vi "BJT_CE_Characterization.vi"() -> ()   [LabVIEW 2020]
panel:
  in  "Tab Control":enum32{"Plot", "Readings", "Information"}(tab)
  out "Temperature / Deg C °":dbl(slide) scale=0.0..100.0
  out "IV Characteristics":cluster{dbl[], dbl[]}[](graph)
  in  "?":bool
  in  "UB":dbl[](array[numeric])=[0.9, 1.0, 1.1, 1.2, 1.3]
  out "UCE":dbl format="%#_3f"
  out "IC":dbl
  out "URC":dbl format="%#_3f"
  out "Numeric":i32
  out "UB/V":dbl
  out "URB/V":dbl format="%#_2f"
  out "UBE/V":dbl format="%#_2f"
  out "UC / V":dbl format="%#_3f"
  out "IB / mA":dbl format="%#_2f"
  # "BJT Values"
  # "IC max = 100 mA"
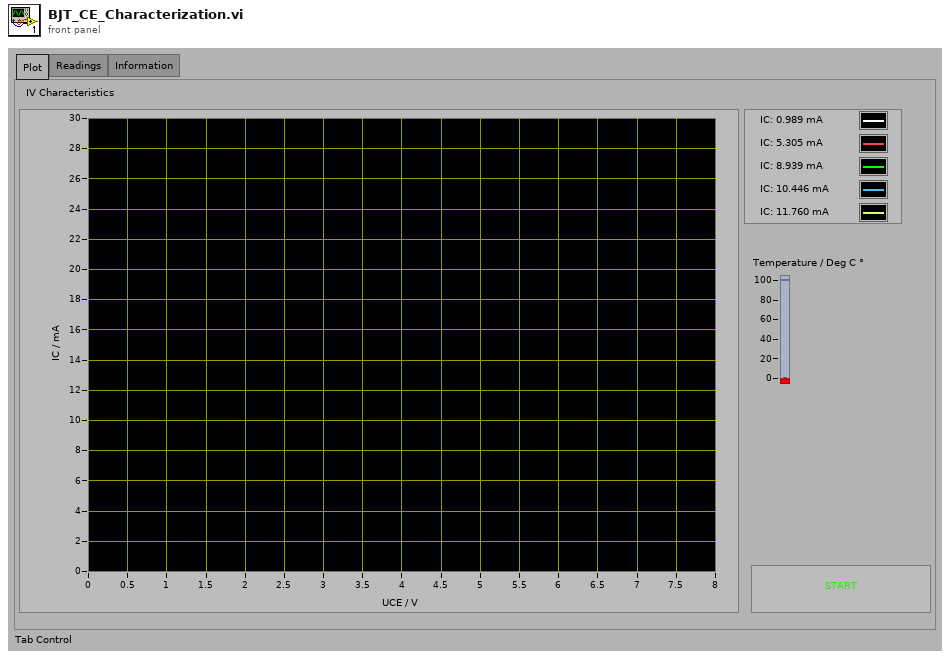
[diagram p1: front panel]
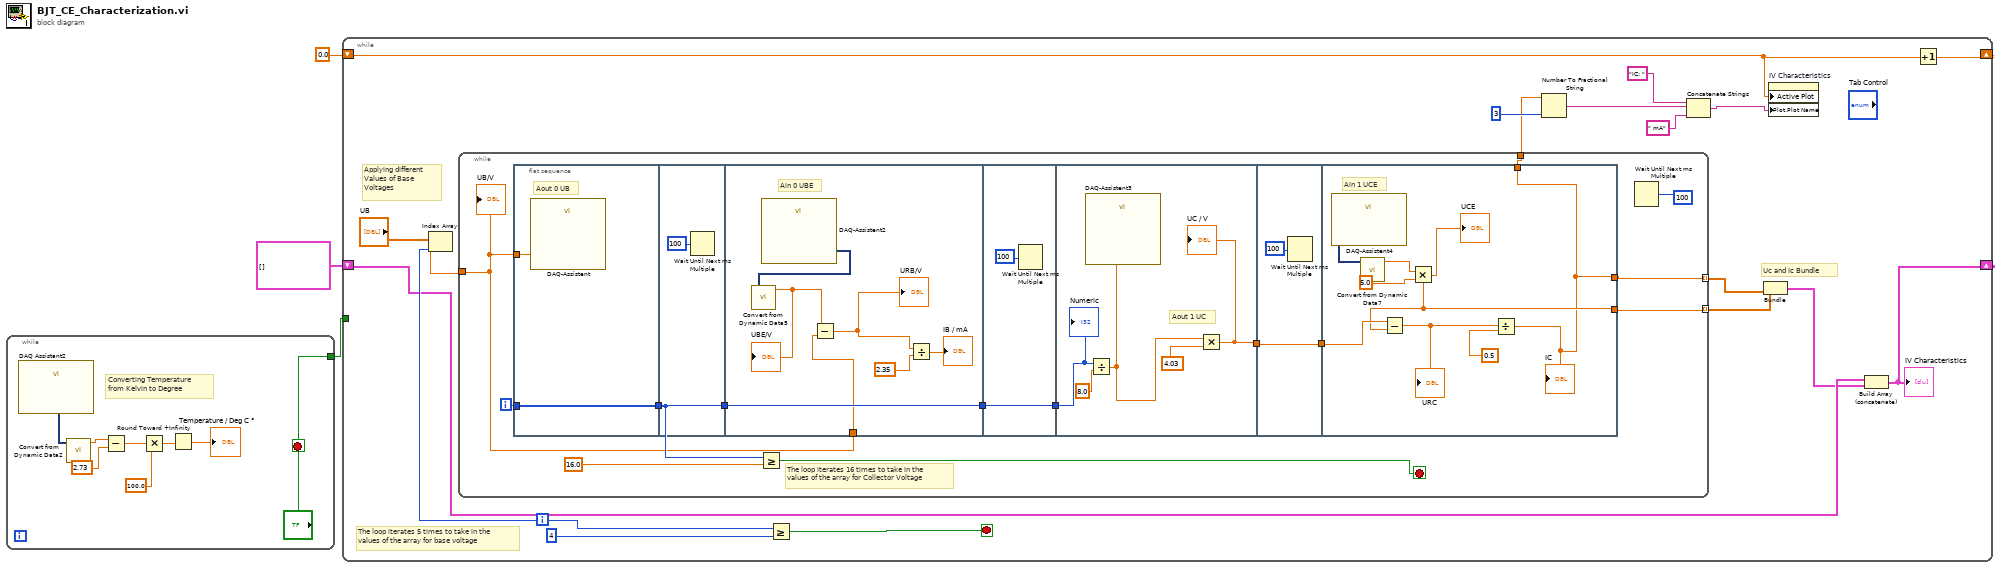
[diagram p0: block diagram]
diagram:
  n1 = while {
    tunnel: ["?"] -> w3
    stop <- "?" stop-if-true
    # "Converting Temperature \nfrom Kelvin to Degree"
    n2 = call "DAQ Assistant2"() -> ("data"=w6:dynamicdata)  [unwired: 17 in, 2 out]
    n3 = call "Convert from Dynamic Data2"("Dynamic Data Type"=w6) -> ("Scalar"=w11:dbl)  [unwired: 3 in]
    n4 = Subtract(x=w11, y=2.73) -> (x-y=w10:dbl)
    n5 = Multiply(x=w10, y=100.0) -> (x*y=w7:dbl)
    n6 = Round Toward +Infinity(x=w7) -> (ceil(x): smallest int >= x=→"Temperature / Deg C °":dbl)
  }
  n7 = while {
    tunnel: w3 -> [_]
    shift-right: [w24] -> _
    shift-left: 0.0 -> [w18]
    shift-right: [w17] -> _
    shift-left: cluster{dbl[], dbl[]}[] [] -> [w16]
    i -> [w27]
    stop <- w28 stop-if-true
    # "Applying different\nValues of Base \nVoltages"
    # "The loop iterates 5 times to take in the \nvalues of the array for base voltage"
    # "Uc and Ic Bundle"
    n8 = Index Array(array="UB", index=w27) -> (element=w29:dbl)
    n9 = while {
      tunnel: w29 -> [w38]
      tunnel: [w36] -> w20
      tunnel: [w35] -> w12 mode=indexing
      tunnel: [w33] -> w13 mode=indexing
      i -> [w41]
      stop <- w43 stop-if-true
      # "The loop iterates 16 times to take in the \nvalues of the array for Collector Voltage"
      n10 = flat-sequence {
        tunnel: w38 -> [w45]
        tunnel: [w44] -> w40
        tunnel: w41 -> [w44]
        tunnel: w40 -> [w47]
        tunnel: [w47] -> w39
        tunnel: w39 -> [w54]
        tunnel: [w54] -> w32
        tunnel: w38 -> [w50]
        tunnel: w32 -> [w56]
        tunnel: [w56] -> w31
        tunnel: w31 -> [w60]
        tunnel: [w57] -> w34
        tunnel: w34 -> [w62]
        tunnel: [w62] -> w30
        tunnel: [w64] -> w36
        tunnel: [w66] -> w35
        tunnel: w30 -> [w67]
        tunnel: [w64] -> w33
        frame #0 {
          # "Aout 0 UB"
          n11 = call "DAQ-Assistent"("data"=w45) -> ()  [unwired: 17 in, 2 out]
        }
        frame #1 {
          n12 = Wait Until Next ms Multiple(millisecond multiple=u32 100) -> ()  [unwired: 1 out]
        }
        frame #2 {
          # "Ain 0 UBE"
          n13 = call "DAQ-Assistent2"() -> ("data"=w52:dynamicdata)  [unwired: 17 in, 2 out]
          n14 = call "Convert from Dynamic Data5"("Dynamic Data Type"=w52) -> ("Scalar"=w53:dbl)  [unwired: 1 in, 2 out]
          "UBE/V" <- w53
          n15 = Subtract(x=w53, y=w50) -> (x-y=w49:dbl)
          "URB/V" <- w49
          n16 = Divide(x=w49, y=2.35) -> (x/y=→"IB / mA":dbl)
        }
        frame #3 {
          n17 = Wait Until Next ms Multiple(millisecond multiple=u32 100) -> ()  [unwired: 1 out]
        }
        frame #4 {
          # "Aout 1 UC"
          n18 = Divide(x=w60, y=8.0) -> (x/y=w58:dbl)
          n19 = call "DAQ-Assistent3"("data"=w58) -> ()  [unwired: 17 in, 2 out]
          n20 = Multiply(x=w58, y=4.03) -> (x*y=w57:dbl)
          "UC / V" <- w57
          "Numeric" <- w60
        }
        frame #5 {
          n21 = Wait Until Next ms Multiple(millisecond multiple=u32 100) -> ()  [unwired: 1 out]
        }
        frame #6 {
          # "Ain 1 UCE"
          n22 = call "DAQ-Assistent4"() -> ("data"=w65:dynamicdata)  [unwired: 17 in, 2 out]
          n23 = call "Convert from Dynamic Data7"("Dynamic Data Type"=w65) -> ("Scalar"=w71:dbl)  [unwired: 1 in, 2 out]
          n24 = Multiply(x=w71, y=5.0) -> (x*y=w66:dbl)
          "UCE" <- w66
          n25 = Subtract(x=w67, y=w66) -> (x-y=w69:dbl)
          "URC" <- w69
          n26 = Divide(x=w69, y=0.5) -> (x/y=w64:dbl)
          "IC" <- w64
        }
      }
      n27 = Greater Or Equal?(x=w41, y=16.0) -> (x >= y?=w43:bool)
      n28 = Wait Until Next ms Multiple(millisecond multiple=u32 100) -> ()  [unwired: 1 out]
      "UB/V" <- w38
    }
    n29 = Greater Or Equal?(x=w27, y=4) -> (x >= y?=w28:bool)
    n30 = Number To Fractional String(number=w20, precision (6)=i16 3) -> (F-format string=w22:string)  [unwired: 2 in]
    n31 = Concatenate Strings("IC: " ("string"), w22, " mA" ("string")) -> (w19:string)
    n32 = Bundle(w12, w13) -> (w15:cluster{dbl[], dbl[]})  [unwired: 1 in]
    n33 = property on="IV Characteristics" class="XYGraph (strict)"("Active Plot"=w18, "Plot.Plot Name"=w19) -> ()  [unwired: 2 in, 2 out]
    n34 = Build Array (concatenate)(w16, w15) -> (w17:cluster{dbl[], dbl[]}[])
    "IV Characteristics" <- w17
    n35 = Increment(x=w18) -> (x+1=w24:dbl)
  }
